vi "PlaceBallSkill.vi"(8 "error in (no error)":errorcluster, 9 "Game":refnum<class "Game.lvclass">, 10 "Robot":refnum<class "Robot.lvclass">, 11 "PlaceBallSkill in":refnum<class "PlaceBallSkill.lvclass">) -> (0 "error out":errorcluster, 1 "finishedPlaceBall":bool, 2 "Robot out":refnum<class "Robot.lvclass">, 3 "PlaceBallSkill out":refnum<class "PlaceBallSkill.lvclass">)   [LabVIEW 2021, in "PlaceBallSkill.lvclass"]
uses:
  PlaceBallSkill.lvclass
  Robot_class/Robot.lvclass
  D:/RoboIme/horie/SSL_AI/Object_class/Object.lvclass
  Game_class/Game.lvclass
  Game_class/Game.lvclass/Game.ctl
  Ball_class/Ball.lvclass/Ball.ctl
  Object_class/Object.lvclass/Object.ctl
  Robot_class/Robot.lvclass/Robot.ctl
  <vilib>/Analysis/_algsub.llb/Real Vector Norm.vi
  <vilib>/Analysis/baseanly.llb/Unit Vector (DBL).vi
  <vilib>/Analysis/coordinate.llb/Wrap Angle (scalar).vi
  Object_class/Read position(x,y).vi
  Robot_class/Read orientation.vi
  Game_class/Read Parameters.lvclass.vi
  Game_class/Read Referee.vi
  Game_class/Read BallRef.vi
  Ball_class/Read v_x.vi
  Ball_class/Read v_y.vi
  Robot_class/Write dest_x.vi
  Robot_class/Write dest_y.vi
  Robot_class/Write dribble.vi
  Robot_class/Write dest_orientation.vi
  Parameters_class/Parameters.lvclass
  Referee_class/Referee.lvclass
  Ball_class/Ball.lvclass
  <vilib>/Analysis/NI_AALBase.lvlib
  Utilities_class/Utilities.lvclass
  <vilib>/Analysis/NI_AAL_Angle.lvlib
  <vilib>/Analysis/NI_AALPro.lvlib
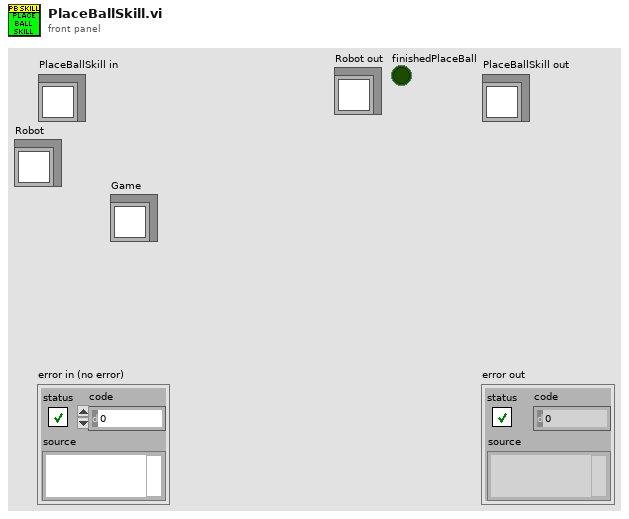
[diagram p1: front panel]
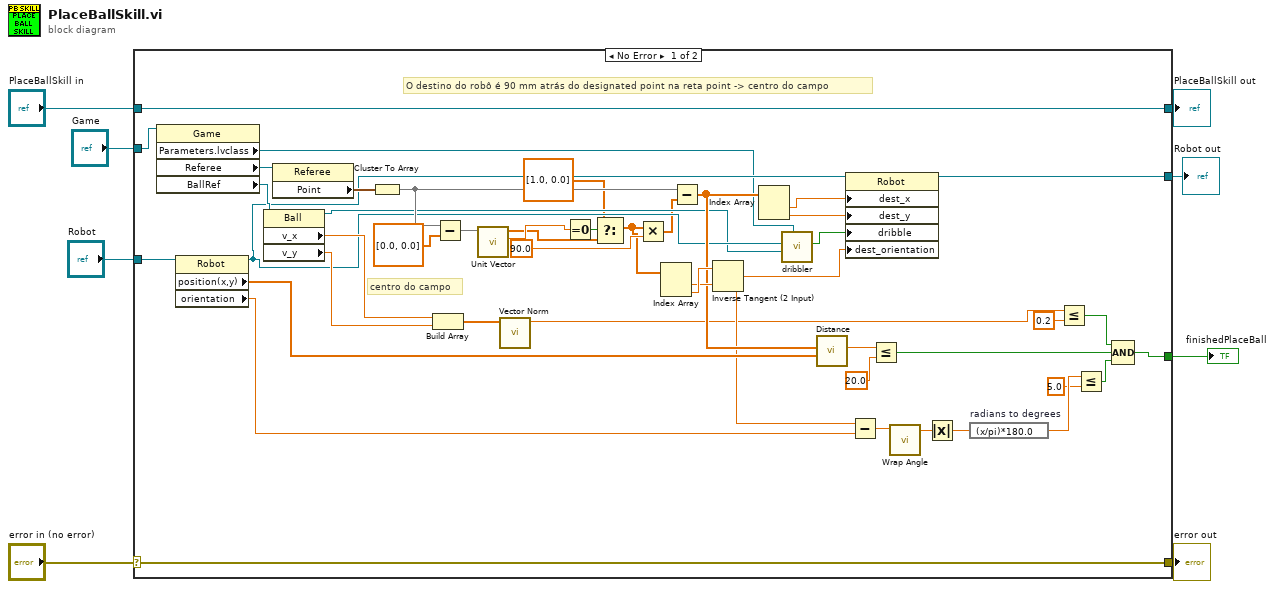
[diagram p0: block diagram]
diagram:
  n1 = case shown="No Error" "error in (no error)" {
    selector: "error in (no error)" -> [w53 w56]
    tunnel: [w53 w56] -> w7
    tunnel: [w54 w55] -> w5
    tunnel: "PlaceBallSkill in" -> [w54 w55]
    tunnel: "Game" -> [w52 _]
    tunnel: "Robot" -> [w49 _]
    tunnel: [w47 _] -> w2
    tunnel: [w28 _] -> w1
    frame No Error {
      # "O destino do robô é 90 mm atrás do designated point na reta point -> centro do campo"
      # "centro do campo"
      n2 = property class="Game"(reference=w52) -> ("Parameters.lvclass"=w17:refnum<class "Parameters.lvclass">, "Referee"=w51:refnum<class "Referee.lvclass">, "BallRef"=w27:refnum<class "Ball.lvclass">)  [unwired: 1 in, 2 out]
      n3 = property class="Robot"(reference=w49) -> (reference out=w19:refnum<class "Robot.lvclass">, "position(x,y)"=w40:dbl[], "orientation"=w35:dbl)  [unwired: 1 in, 1 out]
      n4 = property class="Ball"(reference=w27) -> (reference out=w18:refnum<class "Ball.lvclass">, "v_x"=w26:dbl, "v_y"=w25:dbl)  [unwired: 1 in, 1 out]
      n5 = property class="Referee"(reference=w51) -> ("Point"=w50:cluster{"x":sgl, "y":sgl})  [unwired: 1 in, 2 out]
      n6 = Cluster To Array(cluster=w50) -> (array=w48:sgl[])
      n7 = Build Array(w26, w25) -> (w24:dbl[])
      n8 = Subtract(x=w48, y=sgl[] [0.0, 0.0]) -> (x-y=w44:sgl[])
      n9 = call-poly <vilib>:"Unit Vector.vi"("Input Vector"=w44) -> ("norm"=w15:dbl, "Unit Vector"=w10:dbl[])  [unwired: 8 in, 1 out]
      n10 = call-poly <vilib>:"Vector Norm.vi"("Input Vector"=w24) -> ("norm"=w23:dbl)  [unwired: 9 in, 1 out]
      n11 = Equal To 0?(x=w15) -> (x = 0?=w14:bool)
      n12 = Select(t=dbl[] [1.0, 0.0], s=w14, f=w10) -> (s? t:f=w9:dbl[])
      n13 = Multiply(x=w9, y=90.0) -> (x*y=w11:dbl[])
      n14 = Index Array(array=w9) -> (element #1=w42:dbl, element #2=w43:dbl)  [unwired: 2 in]
      n15 = Subtract(x=w48, y=w11) -> (x-y=w41:dbl[])
      n16 = Inverse Tangent (2 Input)(1:w42, 2:w43) -> (0:w36:dbl)
      n17 = Index Array(array=w41) -> (element #1=w46:dbl, element #2=w45:dbl)  [unwired: 2 in]
      n18 = call "dribbler.vi"("Parameters.lvclass"=w17, "Ball"=w18, "Robot"=w19) -> ("Dribbler?"=w20:bool)  [unwired: 6 in, 2 out]
      n19 = call "Distance.vi"("P1"=w40, "P2"=w41) -> ("Distance"=w39:dbl)  [unwired: 7 in, 2 out]
      n20 = property class="Robot"(reference=w19, "dest_x"=w46, "dest_y"=w45, "dribble"=w20, "dest_orientation"=w36) -> (reference out=w47:refnum<class "Robot.lvclass">)  [unwired: 1 in, 1 out]
      n21 = Subtract(x=w36, y=w35) -> (x-y=w34:dbl)
      n22 = Less Or Equal?(x=w39, y=20.0) -> (x <= y?=w37:bool)
      n23 = call-poly <vilib>:"Wrap Angle.vi"("angle in"=w34) -> ("angle out"=w33:dbl)  [unwired: 9 in, 1 out]
      n24 = Absolute Value(x=w33) -> (abs(x)=w32:dbl)
      n25 = expression code="(x/pi)*180.0" "radians to degrees"(w32) -> (w31:dbl)
      n26 = Less Or Equal?(x=w23, y=0.2) -> (x <= y?=w21:bool)
      n27 = Less Or Equal?(x=w31, y=5.0) -> (x <= y?=w30:bool)
      n28 = Compound Arithmetic op=AND(w21, w37, w30) -> (w28:bool)
    }
    frame Error {
    }
  }
  "error out" <- w7
  "PlaceBallSkill out" <- w5
  "Robot out" <- w2
  "finishedPlaceBall" <- w1
